vi "MFLI -- publish -- dynamic_event.vi"(7 "publisher action":T1, 11 "dynamic event":refnum<user-event>) -> (3 "dynamic event OUT":refnum<user-event>)   [LabVIEW 2018]
uses:
  publisher action.ctl
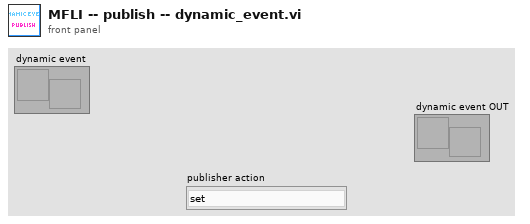
[diagram p1: front panel]
types:
  T1 = typedef "publisher action.ctl" = enum16{"set", "get", "init", "check"}
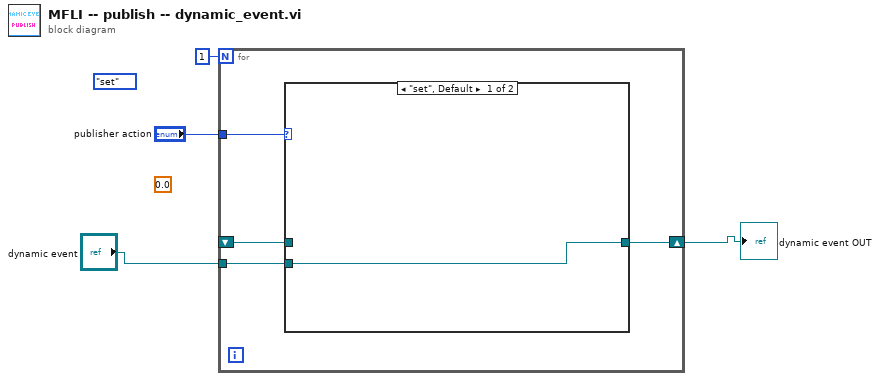
[diagram p0: block diagram]
diagram:
  (unwired) 0.0
  (unwired) publisher_action."set" ("publisher action")
  n1 = for {
    N: 1 -> [_]
    tunnel: "publisher action" -> [w8]
    shift-right: [w7] -> w1
    shift-left: _ -> [w5]
    tunnel: "dynamic event" -> [w6]
    n2 = case shown="\"set\", Default" w8 {
      tunnel: [w9 w10] -> w7
      tunnel: w6 -> [w9 _]
      tunnel: w5 -> [_ w10]
      frame "set", Default {
      }
      frame "get" {
      }
    }
  }
  "dynamic event OUT" <- w1
